vi "Draw Trajectory.vi"(7 "Robot Index":i32, 9 "new picture in":picture, 10 "Trajectory Data":T2(array[cluster]), 11 "Picture in":refnum<vi>) -> (0 "Path Points":cluster{"x":dbl, "y":dbl}[](array[cluster]), 2 "Output Point":T1, 3 "new picture":picture)   [LabVIEW 2020]
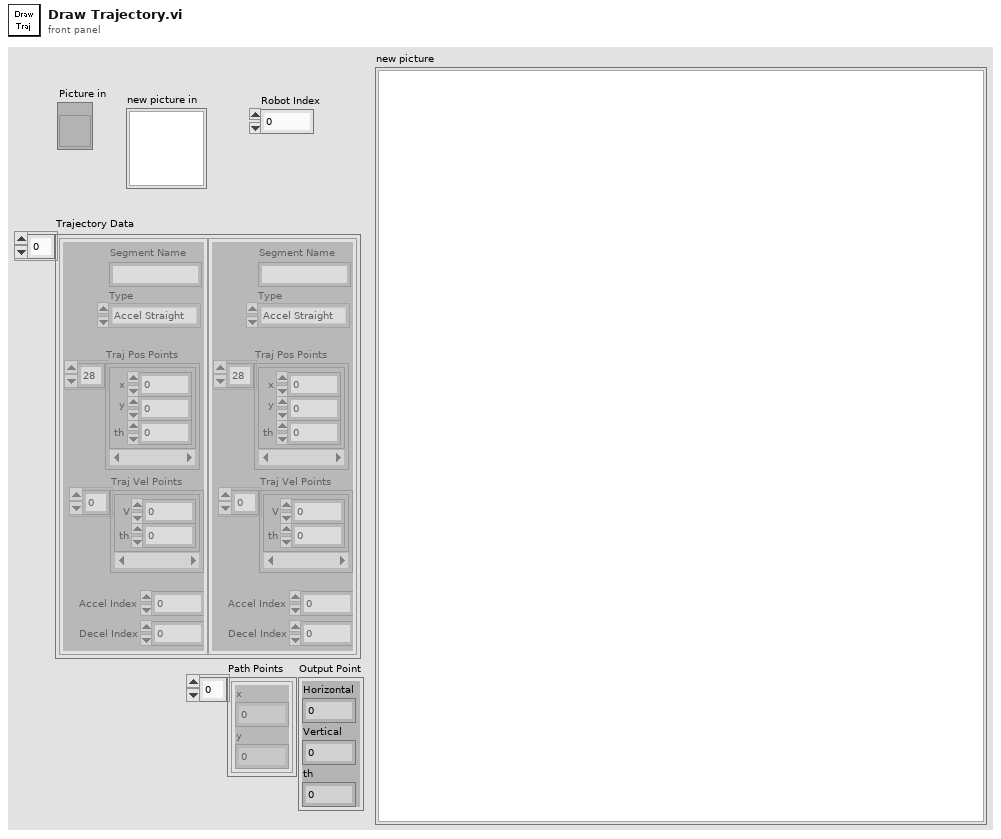
[diagram p1: front panel]
types:
  T1 = cluster{"Horizontal":dbl, "Vertical":dbl, "th":dbl}
  T2 = cluster{"Segment Name":string, "Type":enum16{"Accel Straight", "Const Straight", "Blend", "Circle"}, "Traj Pos Points":cluster{"x":dbl, "y":dbl, "th":dbl}[], "Traj Vel Points":cluster{"V":dbl, "th":dbl}[], "Accel Index":i32, "Decel Index":i32}[]
  T3 = cluster{"Width":u16, "Style":enum32{"Solid", "Dash", "Dot", "DashDot", "DashDotDot"}}
  T4 = typedef "LVPositionTypeDef.ctl" = cluster{"Left":i32, "Top":i32}
  T5 = typedef "LVBoundsTypeDef.ctl" = cluster{"Width":u32, "Height":u32}
  T6 = enum16{"Accel Straight", "Const Straight", "Blend", "Circle"}
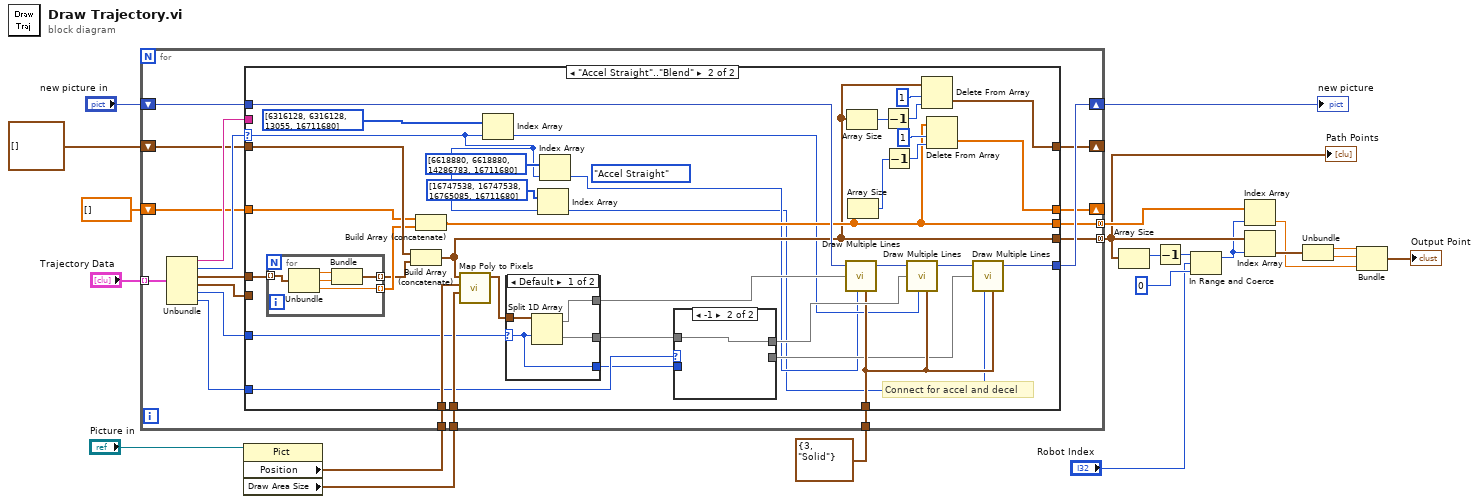
[diagram p0: block diagram]
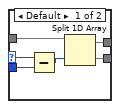
[diagram p3: hidden frame]
diagram:
  n1 = property on="Property Node" class="Pict"(reference="Picture in") -> ("Position"=w16:T4, "Draw Area Size"=w17:T5)  [unwired: 1 in, 2 out]
  n2 = for {
    tunnel: "Trajectory Data" -> [w39] mode=indexing
    shift-right: [w32] -> w15
    shift-left: "new picture in" -> [w31]
    tunnel: T3 {"Width"=3, "Style"=enum."Solid"} ("pen") -> [w35]
    tunnel: w17 -> [w34]
    tunnel: w16 -> [w33]
    tunnel: [w29] -> w8 mode=concatenating
    tunnel: [w28] -> w9 mode=concatenating
    shift-right: [w26] -> _
    shift-left: cluster{"x":dbl, "y":dbl}[] [] -> [w25]
    shift-right: [w24] -> _
    shift-left: dbl[] [] -> [w23]
    n3 = Unbundle(w39) -> ("Segment Name"=w38:string, "Type"=w30:T6, "Traj Pos Points"=w37:cluster{"x":dbl, "y":dbl, "th":dbl}[], "Traj Vel Points"=w36:cluster{"V":dbl, "th":dbl}[], "Accel Index"=w27:i32, "Decel Index"=w22:i32)
    n4 = case shown="\"Accel Straight\"..\"Blend\"" w30 {
      selector: w30 -> [_ w45]
      tunnel: w38 -> [_ _]
      tunnel: w37 -> [_ w79]
      tunnel: w36 -> [_ _]
      tunnel: w35 -> [_ w56]
      tunnel: w34 -> [_ w78]
      tunnel: w33 -> [_ w76]
      tunnel: [w42 w57] -> w32
      tunnel: w31 -> [w42 w77]
      tunnel: [_ w51] -> w29
      tunnel: [_ w65] -> w28
      tunnel: w27 -> [_ w62]
      tunnel: [w41 w70] -> w26
      tunnel: w25 -> [w41 w73]
      tunnel: [w40 w66] -> w24
      tunnel: w23 -> [w40 w63]
      tunnel: w22 -> [_ w61]
      frame Default {
      }
      frame "Accel Straight".."Blend" {
        (unwired) T6."Accel Straight" ("Type")
        # "Connect for accel and decel"
        n5 = for {
          tunnel: w79 -> [w96] mode=indexing
          tunnel: [w95] -> w52 mode=indexing
          tunnel: [w92] -> w64 mode=indexing
          n6 = Unbundle(w96) -> ("x"=w94:dbl, "y"=w93:dbl, "th"=w92:dbl)
          n7 = Bundle("x"=w94, "y"=w93) -> (w95:cluster{"x":dbl, "y":dbl})  [unwired: 1 in]
        }
        n8 = Build Array (concatenate)(w73, w52) -> (w51:cluster{"x":dbl, "y":dbl}[])
        n9 = Build Array (concatenate)(w63, w64) -> (w65:dbl[])
        n10 = call "Map Poly to Pixels.vi"("Draw Area Size"=w78, "Position"=w76, "Coords"=w51) -> ("Coords"=w50:cluster{"Horizontal":dbl, "Vertical":dbl}[])  [unwired: 8 in]
        n11 = Index Array(array=u32[] [6316128, 6316128, 13055, 16711680], index=w45) -> (element=w48:u32)
        n12 = case shown="Default" w62 {
          selector: w62 -> [w87 _]
          tunnel: w50 -> [w90 w91]
          tunnel: [w88 _] -> w49
          tunnel: [w89 w91] -> w54
          tunnel: [w87 _] -> w53
          frame Default {
            n13 = Split 1D Array(array=w90, index=w87) -> (first subarray=w88:cluster{"Horizontal":dbl, "Vertical":dbl}[], second subarray=w89:cluster{"Horizontal":dbl, "Vertical":dbl}[])
          }
          frame -1 {
          }
        }
        n14 = Index Array(array=u32[] [16747538, 16747538, 16765085, 16711680], index=w45) -> (element=w43:u32)
        n15 = Index Array(array=u32[] [6618880, 6618880, 14286783, 16711680], index=w45) -> (element=w44:u32)
        n16 = case shown="-1" w61 {
          selector: w61 -> [w82 _]
          tunnel: w54 -> [w85 w86]
          tunnel: [w84 w86] -> w59
          tunnel: [w83 _] -> w55
          tunnel: w53 -> [w81 _]
          frame Default {
            n17 = Subtract(x=w82, y=w81) -> (x-y=w80:i32)
            n18 = Split 1D Array(array=w85, index=w80) -> (first subarray=w84:cluster{"Horizontal":dbl, "Vertical":dbl}[], second subarray=w83:cluster{"Horizontal":dbl, "Vertical":dbl}[])
          }
          frame -1 {
          }
        }
        n19 = call <vilib>:"Draw Multiple Lines.vi"("picture"=w77, "line endpoints"=w49, "color(black)"=w44, "pen"=w56) -> ("new picture"=w60:picture)  [unwired: 5 in]
        n20 = Array Size(array=w51) -> (size(s)=w74:i32)
        n21 = Array Size(array=w65) -> (size(s)=w67:i32)
        n22 = Decrement(x=w74) -> (x-1=w71:i32)
        n23 = Decrement(x=w67) -> (x-1=w69:i32)
        n24 = call <vilib>:"Draw Multiple Lines.vi"("picture"=w60, "line endpoints"=w59, "color(black)"=w48, "pen"=w56) -> ("new picture"=w58:picture)  [unwired: 5 in]
        n25 = Delete From Array(array=w51, length=1, index=w71) -> (deleted portion=w70:cluster{"x":dbl, "y":dbl}[])  [unwired: 1 out]
        n26 = Delete From Array(array=w65, length=1, index=w69) -> (deleted portion=w66:dbl[])  [unwired: 1 out]
        n27 = call <vilib>:"Draw Multiple Lines.vi"("picture"=w58, "line endpoints"=w55, "color(black)"=w43, "pen"=w56) -> ("new picture"=w57:picture)  [unwired: 5 in]
      }
    }
  }
  "new picture" <- w15
  "Path Points" <- w8
  n28 = Array Size(array=w8) -> (size(s)=w7:i32)
  n29 = Decrement(x=w7) -> (x-1=w6:i32)
  n30 = In Range and Coerce(upper limit=w6, x="Robot Index", lower limit=u16 0 ("Width")) -> (coerced(x)=w3:i32)  [unwired: 1 out]
  n31 = Index Array(array=w9, index=w3) -> (element=w11:dbl)
  n32 = Index Array(array=w8, index=w3) -> (element=w14:cluster{"x":dbl, "y":dbl})
  n33 = Unbundle(w14) -> ("x"=w13:dbl, "y"=w12:dbl)
  n34 = Bundle("x"=w13, "y"=w12, "th"=w11) -> (→"Output Point":cluster{"x":dbl, "y":dbl, "th":dbl})  [unwired: 1 in]
